vi "LVITX ITX2 Plot Commands.vi"(1 "X,Y Log":i32[](array[numeric]), 3 "input string":string="Display/R '#wave#'\nAppendToGraph '#wave#'\nLabel bottom \"#labelX#\"\nLabel left \"#labelY#\"\nModifyGraph rgb('#wave#')=(#r#,#g#,#b#)\n\\\\s('#wave#') #label#\nModifyGraph mirror(bottom)=1\nModifyGraph width=216\nModifyGraph height={Aspect,0.6}\nModifyGraph Log(bottom)=#bottomlog#\nModifyGraph Log(left)=#leftlog#", 4 "Plot labels":string[](array[string])=["time", "V", "V^2", "V^3"], 5 "X,Y Labels":string[](array[string])=["x label", "y label"], 6 "wavenames":string[](array[string])=["time.datatest.000005", "V.datatest.000005", "V^2.datatest.000005", "V^3.datatest.000005"]) -> (0 "result string":string="Display/R 'time.datatest.000005'\nAppendToGraph 'V.datatest.000005'\nAppendToGraph 'V^2.datatest.000005'\nAppendToGraph 'V^3.datatest.000005'\nLabel bottom \"x label\"\nLabel left \"y label\"\nModifyGraph rgb('time.datatest.000005')=(65280,0,0)\nModifyGraph rgb('V.datatest.000005')=(41984,65280,0)\nModifyGraph rgb('V^2.datatest.000005')=(0,65280,45568)\nModifyGraph rgb('V^3.datatest.000005')=(2048,0,65280)\nLegend/C/N=text0/J \"\\\\s('time.datatest.000005') time\\r\\\\s('V.datatest.000005') V\\r\\\\s('V^2.datatest.000005') V^2\\r\\\\s('V^3.datatest.000005') V^3\"\nModifyGraph mirror=1\nModifyGraph width=216\nModifyGraph height={Aspect,0.6}\nModifyGraph Log(bottom)=0\nModifyGraph Log(left)=0\n")   [LabVIEW 2011]
panel:
  # "Legend/C/N=text0/J \"\\\\s('y_test.000011Plot9') Plot 9\\r\\\\s('y_test.000011Plot8') Plot 8\""
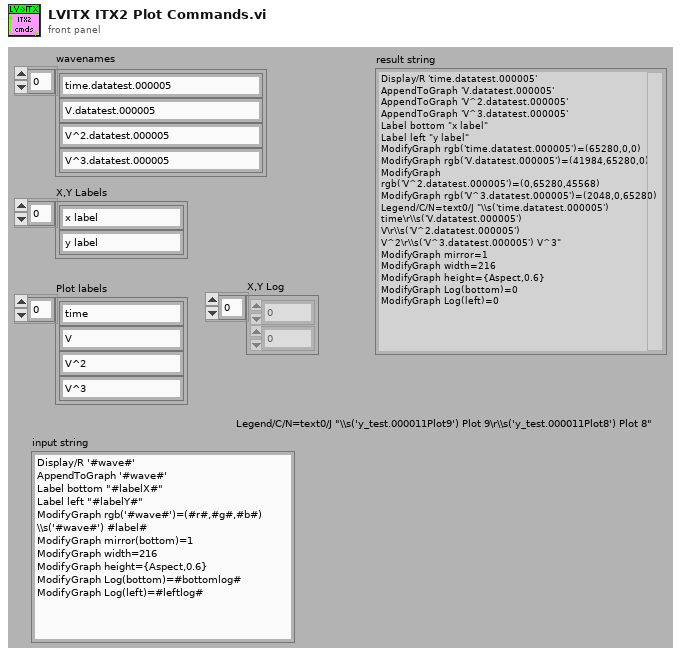
[diagram p1: front panel]
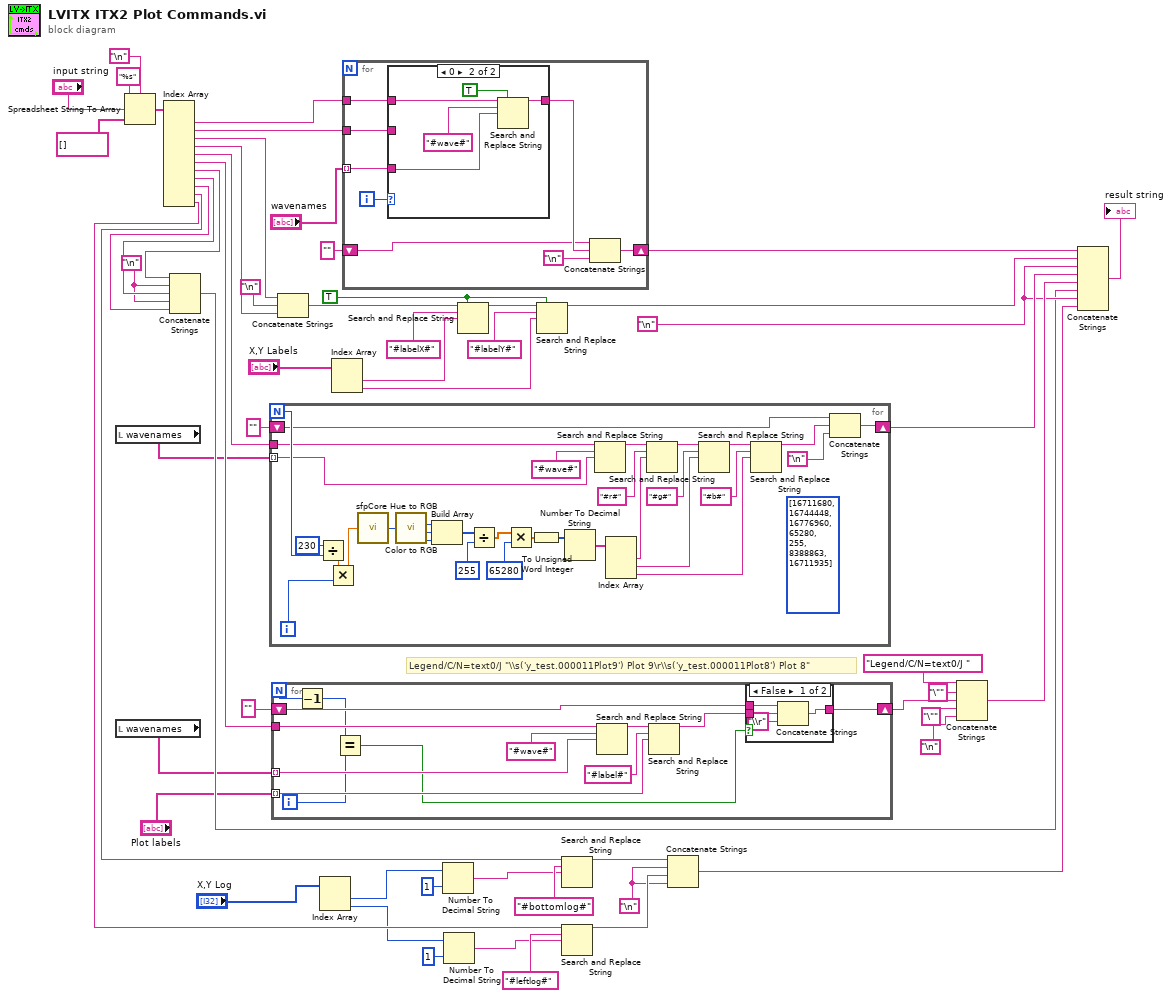
[diagram p0: block diagram]
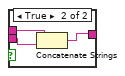
[diagram p2: hidden frame]
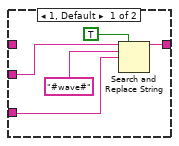
[diagram p3: hidden frame]
diagram:
  w11 = "\n"
  w21 = "\n"
  w20 = "\n"
  w42 = TRUE ("replace all? (F)")
  # "Legend/C/N=text0/J \"\\\\s('y_test.000011Plot9') Plot 9\\r\\\\s('y_test.000011Plot8') Plot 8\""
  n1 = local read "wavenames"() -> (w15:string[])
  n2 = local read "wavenames"() -> (w16:string[])
  n3 = Spreadsheet String To Array(delimiter (Tab)="\n", format string="%s", spreadsheet string="input string", array type (2D Dbl)=string[] []) -> (array=w51:string[])
  n4 = Index Array(array=w51) -> (element #1=w50:string, element #2=w49:string, element #3=w34:string, element #4=w35:string, element #5=w36:string, element #6=w32:string, element #7=w31:string, element #8=w30:string, element #9=w22:string, element #10=w9:string, element #11=w8:string)  [unwired: 11 in]
  n5 = Concatenate Strings(w31, w21, w30, w21, w22) -> (w19:string)
  n6 = for {
    N -> [w79]
    tunnel: w36 -> [w74]
    tunnel: w15 -> [w68] mode=indexing
    shift-right: [w71] -> w40
    shift-left: "" -> [w70]
    i -> [w78]
    (unwired) u32[] [16711680, 16744448, 16776960, 65280, 255, 8388863, 16711935]
    n7 = Divide(x=230, y=w79) -> (x/y=w81:dbl)
    n8 = Multiply(x=w81, y=w78) -> (x*y=w77:dbl)
    n9 = call <userlib>:"sfpCore Hue to RGB.vi"("hue value"=w77) -> ("output color"=w83:u32)
    n10 = call <vilib>:"Color to RGB.vi"("Color"=w83) -> ("R"=w88:u8, "G"=w89:u8, "B"=w90:u8)  [unwired: 1 out]
    n11 = Build Array(w88, w89, w90) -> (w87:u8[])
    n12 = Divide(x=w87, y=255) -> (x/y=w82:dbl[])
    n13 = Multiply(x=w82, y=65280) -> (x*y=w84:dbl[])
    n14 = To Unsigned Word Integer(number=w84) -> (unsigned 16bit integer=w76:u16[])
    n15 = Number To Decimal String(number=w76) -> (decimal integer string=w63:string[])  [unwired: 1 out]
    n16 = Search and Replace String(input string=w74, search string="#wave#", replace string=w68) -> (result string=w75:string)  [unwired: 1 in, 7 out]
    n17 = Index Array(array=w63) -> (element #1=w62:string, element #2=w61:string, element #3=w60:string)  [unwired: 3 in]
    n18 = Search and Replace String(input string=w75, search string="#r#", replace string=w62) -> (result string=w73:string)  [unwired: 1 in, 7 out]
    n19 = Search and Replace String(input string=w73, search string="#g#", replace string=w61) -> (result string=w72:string)  [unwired: 1 in, 7 out]
    n20 = Search and Replace String(input string=w72, search string="#b#", replace string=w60) -> (result string=w67:string)  [unwired: 1 in, 7 out]
    n21 = Concatenate Strings(w70, w67, "\n") -> (w71:string)
  }
  n22 = for {
    N -> [w94]
    shift-right: [w95] -> w25
    shift-left: "" -> [w102]
    tunnel: "Plot labels" -> [w96] mode=indexing
    tunnel: w32 -> [w99]
    tunnel: w16 -> [w98] mode=indexing
    i -> [w92]
    n23 = Decrement(x=w94) -> (x-1=w93:i32)
    n24 = Equal?(x=w93, y=w92) -> (x = y?=w91:bool)
    n25 = Search and Replace String(input string=w99, search string="#wave#", replace string=w98) -> (result string=w103:string)  [unwired: 1 in, 7 out]
    n26 = Search and Replace String(input string=w103, search string="#label#", replace string=w96) -> (result string=w97:string)  [unwired: 1 in, 7 out]
    n27 = case shown="False" w91 {
      tunnel: w102 -> [w107 w109]
      tunnel: w97 -> [w106 w108]
      tunnel: [w105 w110] -> w95
      frame False {
        n28 = Concatenate Strings(w107, w106, "\\r" ("string")) -> (w105:string)
      }
      frame True {
        n29 = Concatenate Strings(w109, w108) -> (w110:string)
      }
    }
  }
  n30 = Concatenate Strings(w34, "\n", w35) -> (w47:string)
  n31 = Index Array(array="X,Y Log") -> (element #1=w2:i32, element #2=w1:i32)  [unwired: 2 in]
  n32 = Index Array(array="X,Y Labels") -> (element #1=w38:string, element #2=w37:string)  [unwired: 2 in]
  n33 = for {
    tunnel: "wavenames" -> [w116] mode=indexing
    tunnel: w50 -> [w118]
    tunnel: w49 -> [w117]
    shift-right: [w114] -> w55
    shift-left: "" -> [w111]
    i -> [w115]
    n34 = case shown="0" w115 {
      tunnel: w118 -> [_ w126]
      tunnel: w117 -> [w121 _]
      tunnel: w116 -> [w122 w127]
      tunnel: [w120 w125] -> w113
      frame 1, Default {
        n35 = Search and Replace String(replace all?=TRUE ("replace all? (F)"), input string=w121, search string="#wave#", replace string=w122) -> (result string=w120:string)  [unwired: 1 in, 6 out]
      }
      frame 0 {
        n36 = Search and Replace String(replace all?=TRUE ("replace all? (F)"), input string=w126, search string="#wave#", replace string=w127) -> (result string=w125:string)  [unwired: 1 in, 6 out]
      }
    }
    n37 = Concatenate Strings(w111, w113, "\n") -> (w114:string)
  }
  n38 = Number To Decimal String(number=w2, width (-)=i16 1) -> (decimal integer string=w4:string)
  n39 = Number To Decimal String(number=w1, width (-)=i16 1) -> (decimal integer string=w5:string)
  n40 = Search and Replace String(replace all?=w42, input string=w47, search string="#labelX#", replace string=w38) -> (result string=w45:string)  [unwired: 1 in, 6 out]
  n41 = Search and Replace String(replace all?=w42, input string=w45, search string="#labelY#", replace string=w37) -> (result string=w33:string)  [unwired: 1 in, 6 out]
  n42 = Search and Replace String(input string=w9, search string="#bottomlog#", replace string=w4) -> (result string=w13:string)  [unwired: 1 in, 7 out]
  n43 = Search and Replace String(input string=w8, search string="#leftlog#", replace string=w5) -> (result string=w12:string)  [unwired: 1 in, 7 out]
  n44 = Concatenate Strings(w13, w11, w12, w11) -> (w10:string)
  n45 = Concatenate Strings("Legend/C/N=text0/J ", "\"" ("string"), w25, "\"" ("string"), "\n") -> (w27:string)
  n46 = Concatenate Strings(w55, w33, w20, w40, w27, w19, w20, w10) -> (→"result string":string)
